vi "Handle Command.vi"(8 "error in (no error)":errorcluster, 9 "Data":variant, 10 "Command":string, 11 "Inst.Framework-Template in":refnum<class "Inst.Framework-Template.lvclass">) -> (0 "error out":errorcluster, 1 "Processed Data":variant, 2 "Command":string, 3 "Inst.Framework-Template out":refnum<class "Inst.Framework-Template.lvclass">)   [LabVIEW 2019, in "Inst.Framework-Template.lvclass"]
uses:
  Inst.Framework-Template.lvclass
  Inst.Framework-Template.lvclass/Inst.Framework-Template.ctl
  9aec49fd-fe04-463a-be35-b7075f22e824.vi
  9aec49fd-fe04-463a-be35-b7075f22e824.vi/abe5fa22-c859-44fd-8cbb-fe953b695161.vi
  9aec49fd-fe04-463a-be35-b7075f22e824.vi/39658901-e9d6-4c0e-9991-2933a94fda44.vi
  <vilib>/Utility/Data Type/Get Type Information.vi
  <vilib>/JDP Science/JSONtext/JSON text to Variant.vi
  <vilib>/JDP Science/JSONtext/LVClass Serializer/JSONtext LVClass Serializer.lvclass
  <userlib>/LevyLab/Instrument Framework/Instrument Types/VSource/Instrument.VSource.lvclass
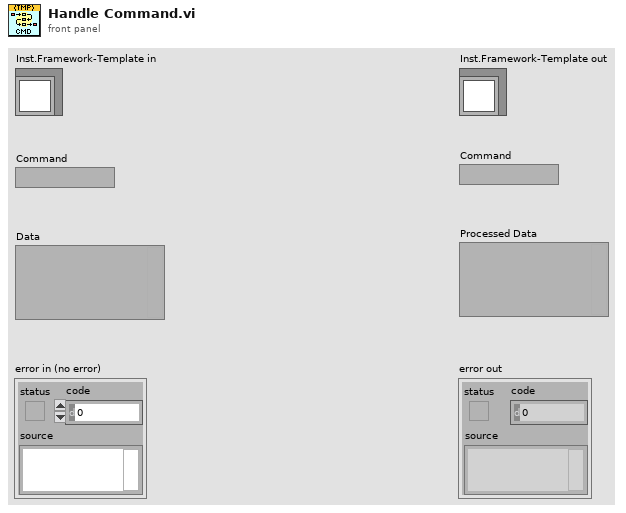
[diagram p1: front panel]
types:
  T1 = typedef "Inst.Framework-Template.lvclass/Inst.Framework-Template.getAll--Cluster.ctl" = cluster{"Levy 1":dbl, "Logger SMO":dbl, "SMO Boolean":bool, "SMO String":string}
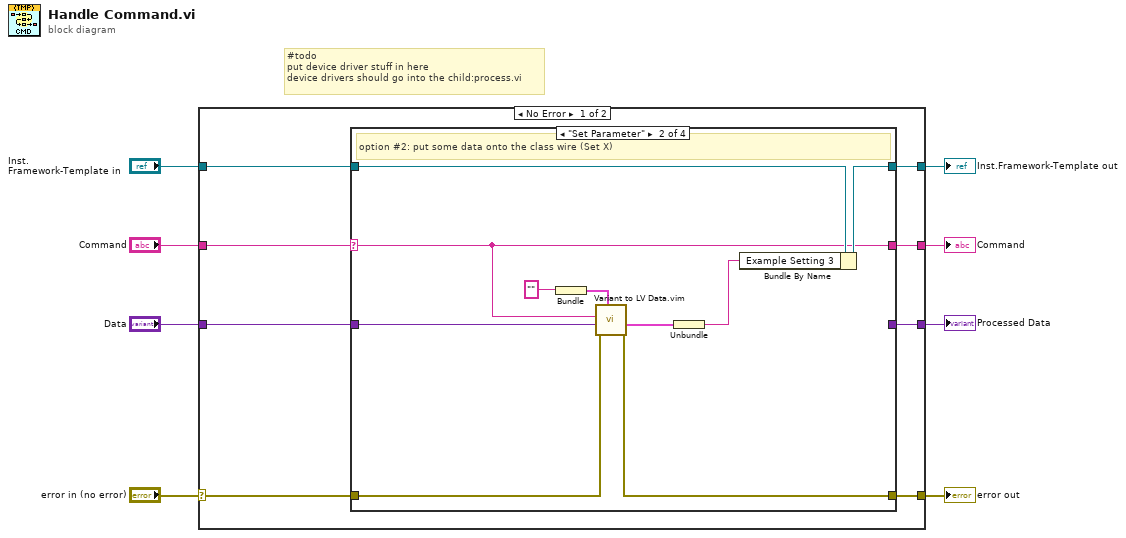
[diagram p0: block diagram]
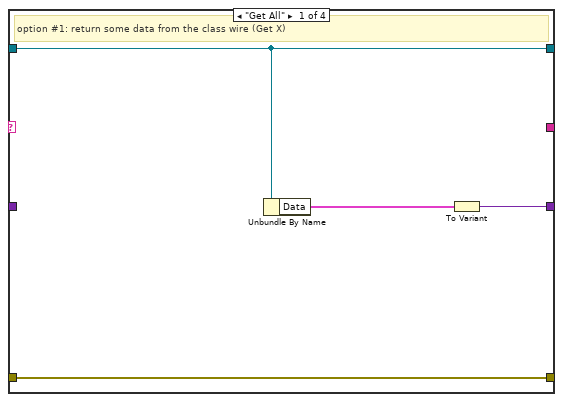
[diagram p2: hidden frame]
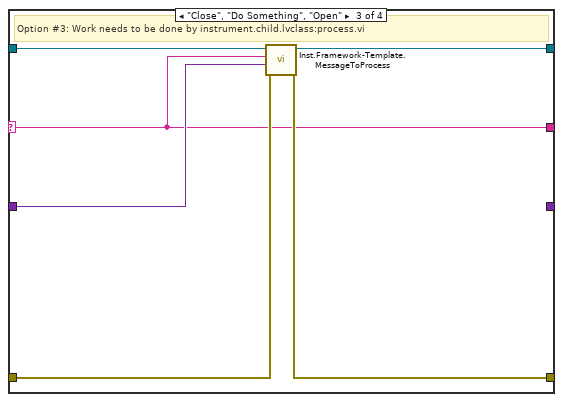
[diagram p3: hidden frame]
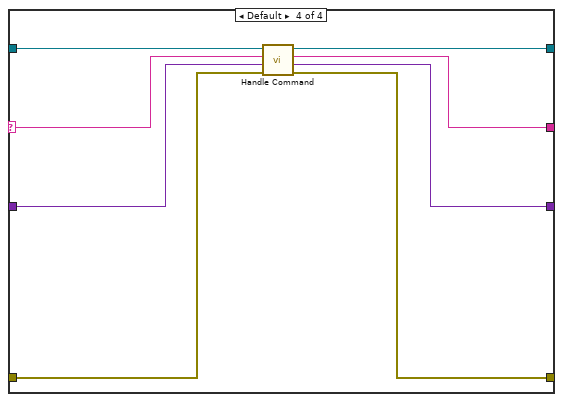
[diagram p4: hidden frame]
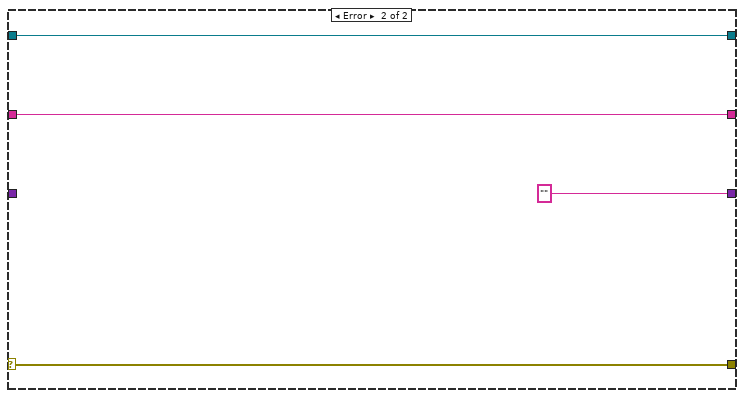
[diagram p5: hidden frame]
diagram:
  # "#todo\nput device driver stuff in here\ndevice drivers should go into the child:process.vi"
  n1 = case shown="No Error" "error in (no error)" {
    selector: "error in (no error)" -> [w10 w48]
    tunnel: [w12 w48] -> w6
    tunnel: [w14 w47] -> w5
    tunnel: "Inst.Framework-Template in" -> [w15 w47]
    tunnel: "Command" -> [w16 w45]
    tunnel: [w13 "" ("String")] -> w3
    tunnel: "Data" -> [w9 _]
    tunnel: [w11 w45] -> w1
    frame No Error {
      n2 = case shown="\"Set Parameter\"" w16 {
        selector: w16 -> [_ w25 w31 w38]
        tunnel: w15 -> [w19 w30 w36 w42]
        tunnel: [w19 w29 w35 w39] -> w14
        tunnel: [w17 _ _ w41] -> w13
        tunnel: w10 -> [w18 w28 w34 w43]
        tunnel: w9 -> [_ w26 w32 w44]
        tunnel: [w18 w27 w33 w40] -> w12
        tunnel: [_ w25 w31 w37] -> w11
        frame "Get All" {
          # "option #1: return some data from the class wire (Get X)"
          n3 = Unbundle By Name(w19) -> ("Data"=w20:T1)
          n4 = To Variant(anything=w20) -> (Variant=w17:variant)
        }
        frame "Set Parameter" {
          # "option #2: put some data onto the class wire (Set X)"
          n5 = Bundle("") -> (w23:cluster{string})  [unwired: 1 in]
          n6 = call "Variant to LV Data.vim"("type"=w23, "error in (no error)"=w28, "JSON Data in"=w26, "Command"=w25) -> ("error out"=w27:errorcluster, "Data out"=w22:cluster{string})  [unwired: 4 in, 2 out]
          n7 = Unbundle(w22) -> (w21:string)
          n8 = Bundle By Name(cluster=w30, "Example Setting 3"=w21) -> (w29:refnum<class "Inst.Framework-Template.lvclass">)
        }
        frame "Close", "Do Something", "Open" {
          # "Option #3: Work needs to be done by instrument.child.lvclass:process.vi"
          n9 = call "Inst.Framework-Template.MessageToProcess.vi"("error in (no error)"=w34, "Data"=w32, "Command"=w31, "Framework-Template in"=w36) -> ("error out"=w33:errorcluster, "Framework-Template out"=w35:refnum<class "Inst.Framework-Template.lvclass">)  [unwired: 6 in]
        }
        frame Default {
          n10 = call-parent "Handle Command.vi"("error in (no error)"=w43, "Data"=w44, "Command"=w38, "Instrument in"=w42) -> ("error out"=w40:errorcluster, "Processed Data"=w41:variant, "Command"=w37:string, "Instrument out"=w39:refnum<class "Inst.Framework-Template.lvclass">)  [unwired: 4 in]
        }
      }
    }
    frame Error {
    }
  }
  "error out" <- w6
  "Inst.Framework-Template out" <- w5
  "Command" <- w1
  "Processed Data" <- w3
